vi "LabJack_init.vi"(8 "error in":errorcluster, 11 "Positive Channel #":i32) -> (0 "error out":errorcluster, 2 "status":bool, 3 "Handle Out":i32)   [LabVIEW 2019]
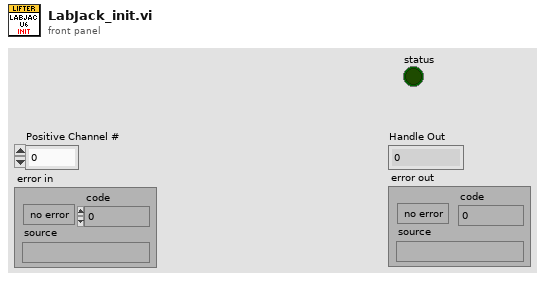
[diagram p1: front panel]
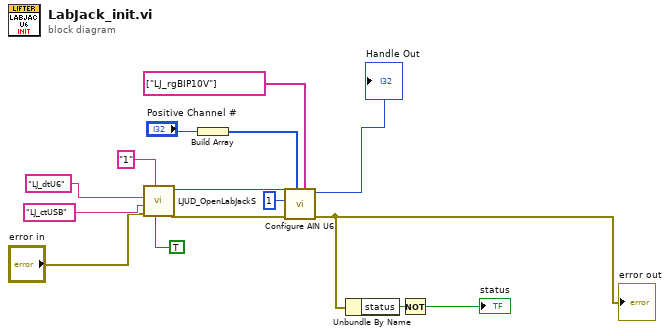
[diagram p0: block diagram]
diagram:
  n1 = call "LJUD_OpenLabJackS.vi"("FirstFound"=TRUE, "Address"="1", "error in"="error in", "ConnectionType"="LJ_ctUSB", "DeviceType"="LJ_dtU6") -> ("error out"=w9:errorcluster, "Handle"=w10:i32)  [unwired: 4 in, 1 out]
  n2 = Build Array("Positive Channel #") -> (w3:i32[])
  n3 = call "Configure AIN U6.vi"("Ranges"=string[] ["LJ_rgBIP10V"], "Positive Channels"=w3, "error in"=w9, "Resolution"=1, "Handle In"=w10) -> ("error out"=w2:errorcluster, "Handle Out"=→"Handle Out":i32)  [unwired: 5 in]
  "error out" <- w2
  n4 = Unbundle By Name(w2) -> ("status"=w7:bool)
  n5 = Not(x=w7) -> (.not. x?=→"status":bool)
